vi "1D_Data_to_Igor_with_Prefix.vi"(6 "Do Transfer":bool=TRUE, 8 "error in (no error)":errorcluster, 9 "Wave Name":string, 10 "Wave Prefix":string, 11 "Data":dbl[](array[numeric])=[88.25201560693692, 88.167918910518, 88.08981318404682, 88.0168868285138, 87.95089009612809, 87.89039736256106, 87.83704227062073, 87.78920015031018, 87.7485542000132, 87.71337659128233, 87.68541510328214, 87.66287703285205, 87.64756317461499, 87.63764334319724, 87.63495129520638, 87.63764334319724, 87.64756317461499, 87.66287703285205, 87.68541510328214, 87.71337659128233, 87.7485542000132, 87.78920015031018, 87.83704227062073, 87.89039736256106, 87.95089009612809, 88.0168868285138, 88.08981318404682, 88.167918910518, 88.25201560693691] format="%.2f") -> (0 "error out":errorcluster, 2 "Wave Prefix Through":string)   [LabVIEW 2010]
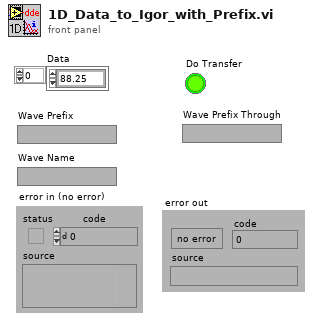
[diagram p1: front panel]
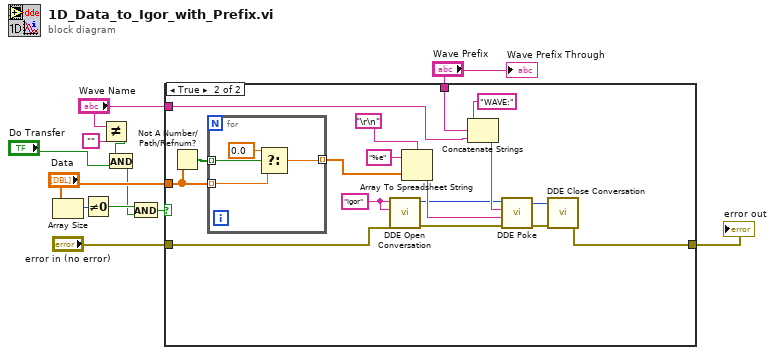
[diagram p0: block diagram]
diagram:
  n1 = Array Size(array="Data") -> (size(s)=w12:i32)
  n2 = Not Equal To 0?(x=w12) -> (x != 0?=w9:bool)
  n3 = Not Equal?(x="Wave Name", y="") -> (x != y?=w2:bool)
  n4 = And(x=w2, y="Do Transfer") -> (x .and. y?=w3:bool)
  n5 = And(x=w9, y=w3) -> (x .and. y?=w10:bool)
  n6 = case shown="True" w10 {
    tunnel: "Data" -> [_ w20]
    tunnel: "Wave Name" -> [_ w16]
    tunnel: "Wave Prefix" -> [_ w19]
    tunnel: "error in (no error)" -> [w13 w17]
    tunnel: [w13 w18] -> w5
    frame False {
    }
    frame True {
      w30 = "Igor" ("service")
      n7 = Not A Number/Path/Refnum?(number/path/refnum=w20) -> (NaN/Path/Refnum?=w23:bool[])
      n8 = for {
        tunnel: w23 -> [w34] mode=indexing
        tunnel: w20 -> [w33] mode=indexing
        tunnel: [w32] -> w22 mode=indexing
        n9 = Select(t=0.0, s=w34, f=w33) -> (s? t:f=w32:dbl)
      }
      n10 = call "DDE Open Conversation.vi"("error in (no error)"=w17, "topic"=w30, "service"=w30) -> ("error out"=w25:errorcluster, "conversation refnum"=w24:u32)  [unwired: 5 in]
      n11 = Array To Spreadsheet String(delimiter (Tab)="\r\n", array=w22, 3:"%e" ("format string")) -> (spreadsheet string=w27:string)
      n12 = Concatenate Strings("WAVE:", w19, w16) -> (w26:string)
      n13 = call "DDE Poke.vi"("error in (no error)"=w25, "data"=w27, "item"=w26, "conversation refnum in"=w24) -> ("error out"=w15:errorcluster, "conversation refnum out"=w14:u32)  [unwired: 4 in]
      n14 = call "DDE Close Conversation.vi"("error in (no error)"=w15, "conversation refnum"=w14) -> ("error out"=w18:errorcluster)  [unwired: 7 in]
    }
  }
  "error out" <- w5
  "Wave Prefix Through" <- "Wave Prefix"
